vi "Disable & Enable.vi"(8 "error in (no error)":errorcluster, 9 "Disabled?":bool, 11 "Control Ref Array":refnum<vi>[](array[refnum])) -> (0 "error out":errorcluster)   [LabVIEW 2017, in "2D Plot.lvclass"]
uses:
  <vilib>/Math Plots/2D Math Plots/2D Plot/2D Plot/2D Plot.lvclass
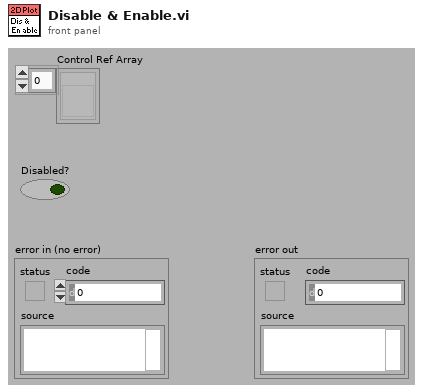
[diagram p1: front panel]
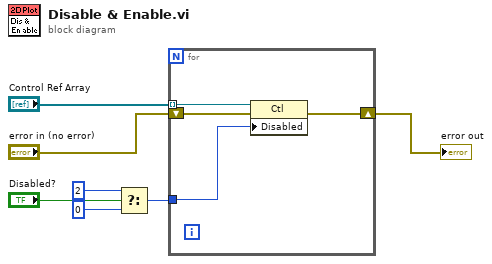
[diagram p0: block diagram]
diagram:
  n1 = Select(t=u8 2 ("Disabled"), s="Disabled?", f=u8 0) -> (s? t:f=w2:u8)
  n2 = for {
    tunnel: "Control Ref Array" -> [w11] mode=indexing
    shift-right: [w10] -> w5
    shift-left: "error in (no error)" -> [w9]
    tunnel: w2 -> [w8]
    n3 = property class="Ctl"(reference=w11, error in=w9, "Disabled"=w8) -> (error out=w10:errorcluster)  [unwired: 1 out]
  }
  "error out" <- w5
